vi "GA_Crossover.vi"(10 "pop[idx]_500":i32[](array[numeric])) -> (0 "pop(500*20) 2":i32[][](array[numeric]), 2 "pop(500*20)":i32[][](array[numeric]))   [LabVIEW 2018]
uses:
  GA_Global.vi
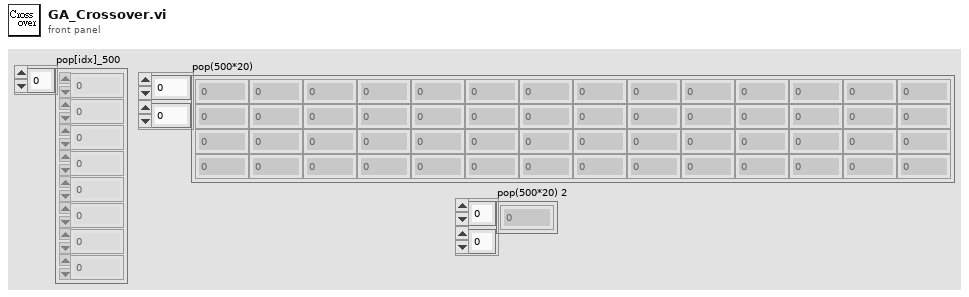
[diagram p1: front panel]
types:
  T1 = typedef "GA_parameter.ctl" = cluster{"N_CITIES":i32, "POP_SIZE":i32, "N_GENERATIONS":i32, "CROSS_RATE":dbl, "MUTATE_RATE":dbl}
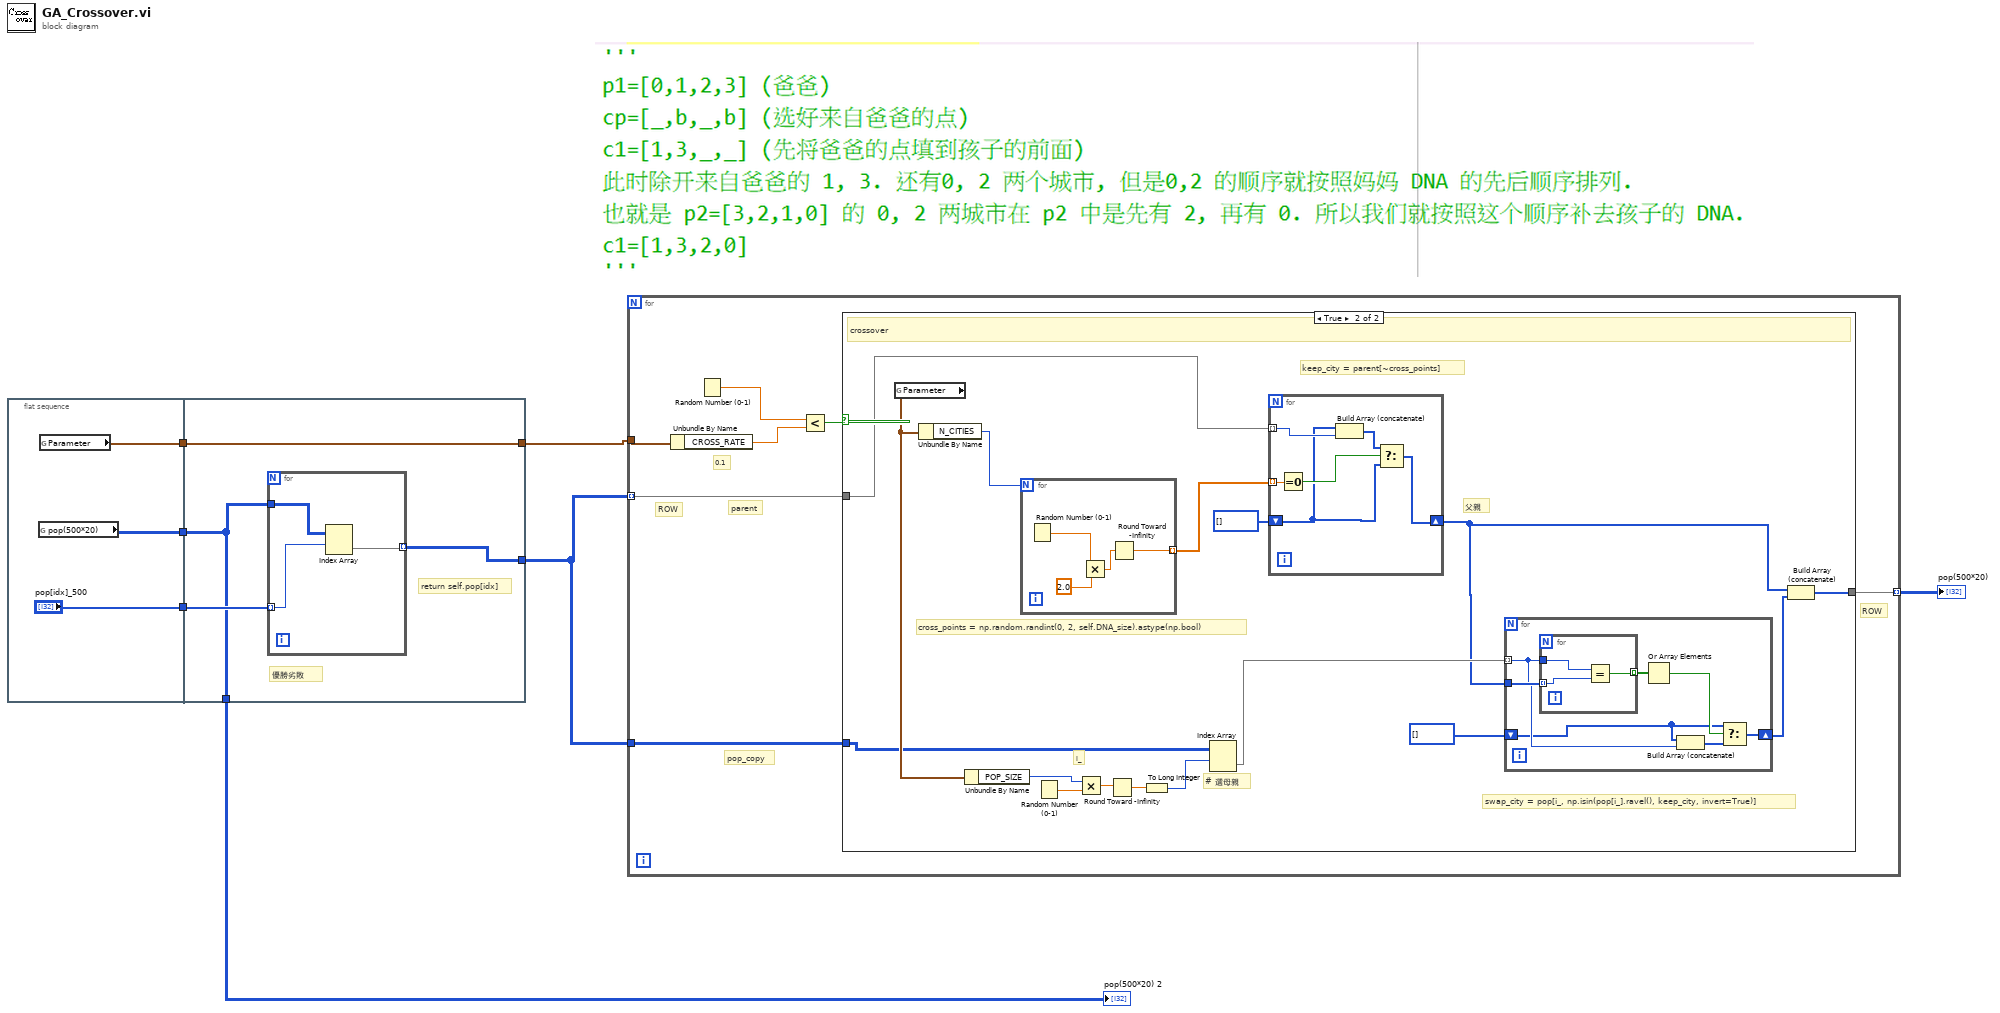
[diagram p0: block diagram]
diagram:
  n1 = flat-sequence {
    tunnel: [w10] -> w5
    tunnel: [w9] -> w4
    tunnel: ["pop[idx]_500"] -> w3
    tunnel: [w14] -> w7
    tunnel: [w12] -> w2
    tunnel: w5 -> [w11]
    tunnel: w4 -> [w14]
    tunnel: w3 -> [w13]
    tunnel: [w11] -> w1
    frame #0 {
      n2 = global read "GA_Global.vi" "pop(500*20)"() -> (w10:i32[][])
      n3 = global read "GA_Global.vi" "Parameter"() -> (w9:T1)
    }
    frame #1 {
      # "優勝劣敗"
      # "return self.pop[idx]"
      n4 = for {
        tunnel: w11 -> [w17]
        tunnel: w13 -> [w16] mode=indexing
        tunnel: [w15] -> w12 mode=indexing
        n5 = Index Array "Index Array"(array=w17, index (row)=w16) -> (element=w15:i32[])  [unwired: 1 in]
      }
    }
  }
  n6 = for {
    tunnel: w2 -> [w20] mode=indexing
    tunnel: w7 -> [w24]
    tunnel: [w19] -> w6 mode=indexing
    tunnel: w2 -> [w18]
    # "0.1"
    # "ROW"
    # "ROW"
    # "pop_copy"
    # "parent"
    n7 = Unbundle By Name(w24) -> ("CROSS_RATE"=w22:dbl)
    n8 = Random Number (0-1)() -> (number: 0 to 1=w23:dbl)
    n9 = Less?(x=w23, y=w22) -> (x < y?=w21:bool)
    n10 = case shown="True" w21 {
      tunnel: w20 -> [w25 w31]
      tunnel: [w25 w32] -> w19
      tunnel: w18 -> [_ w30]
      frame False {
      }
      frame True {
        # "swap_city = pop[i_, np.isin(pop[i_].ravel(), keep_city, invert=True)]"
        # "父親"
        # "# 選母親"
        # "i_"
        # "keep_city = parent[~cross_points]"
        # "cross_points = np.random.randint(0, 2, self.DNA_size).astype(np.bool)"
        # "crossover"
        n11 = global read "GA_Global.vi" "Parameter"() -> (w37:T1)
        n12 = Unbundle By Name(w37) -> ("N_CITIES"=w41:i32)
        n13 = Unbundle By Name(w37) -> ("POP_SIZE"=w36:i32)
        n14 = for {
          N: w41 -> [_]
          tunnel: [w58] -> w33 mode=indexing
          n15 = Random Number (0-1)() -> (number: 0 to 1=w61:dbl)
          n16 = Multiply(x=w61, y=2.0) -> (x*y=w59:dbl)
          n17 = Round Toward -Infinity(1:w59) -> (0:w58:dbl)
        }
        n18 = Random Number (0-1)() -> (number: 0 to 1=w39:dbl)
        n19 = Multiply(x=w36, y=w39) -> (x*y=w38:dbl)
        n20 = Round Toward -Infinity(1:w38) -> (0:w35:dbl)
        n21 = To Long Integer(number=w35) -> (32bit integer=w34:i32)
        n22 = Index Array(array=w30, index (row)=w34) -> (element=w28:i32[])  [unwired: 1 in]
        n23 = for {
          tunnel: w31 -> [w54] mode=indexing
          shift-right: [w55] -> w27
          shift-left: i32[] [] -> [w52]
          tunnel: w33 -> [w57] mode=indexing
          n24 = Equal To 0?(x=w57) -> (x = 0?=w56:bool)
          n25 = Build Array (concatenate)(w52, w54) -> (w53:i32[])
          n26 = Select(t=w53, s=w56, f=w52) -> (s? t:f=w55:i32[])
        }
        n27 = for {
          tunnel: w28 -> [w44] mode=indexing
          tunnel: w27 -> [w48]
          shift-right: [w46] -> w26
          shift-left: i32[] [] -> [w43]
          n28 = for {
            tunnel: w48 -> [w50] mode=indexing
            tunnel: w44 -> [w51]
            tunnel: [w49] -> w47 mode=indexing
            n29 = Equal?(x=w51, y=w50) -> (x = y?=w49:bool)
          }
          n30 = Or Array Elements(Boolean array=w47) -> (logical OR=w45:bool)
          n31 = Build Array (concatenate)(w43, w44) -> (w42:i32[])
          n32 = Select(t=w43, s=w45, f=w42) -> (s? t:f=w46:i32[])
        }
        n33 = Build Array (concatenate)(w27, w26) -> (w32:i32[])
      }
    }
  }
  "pop(500*20)" <- w6
  "pop(500*20) 2" <- w1
